vi "SLL DE Group Device Based on Catagory.vi"(8 "error Input":errorcluster, 9 "Module Dev Names":cluster{"Chassis.ModuleDevNames":tag[]}[](array[cluster]), 10 "Chassis Names":tag[](array[tag]), 11 "Device Names":tag[](array[tag])) -> (0 "error out":errorcluster, 2 "Devices Names":string[](array[string]), 3 "All Device Names (Chassis & Module)":cluster{"New element":tag[]}[](array[cluster]))   [LabVIEW 2013]
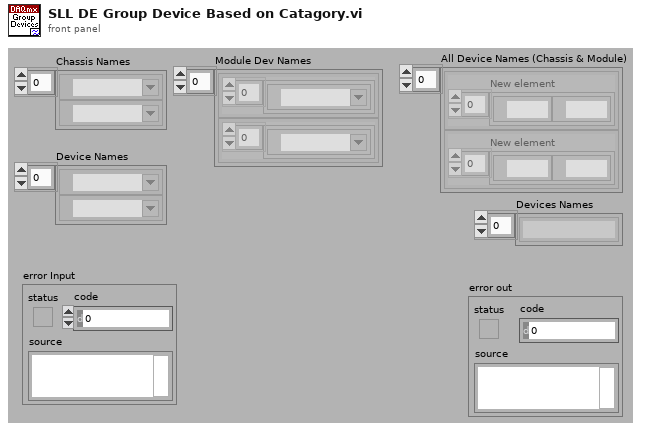
[diagram p1: front panel]
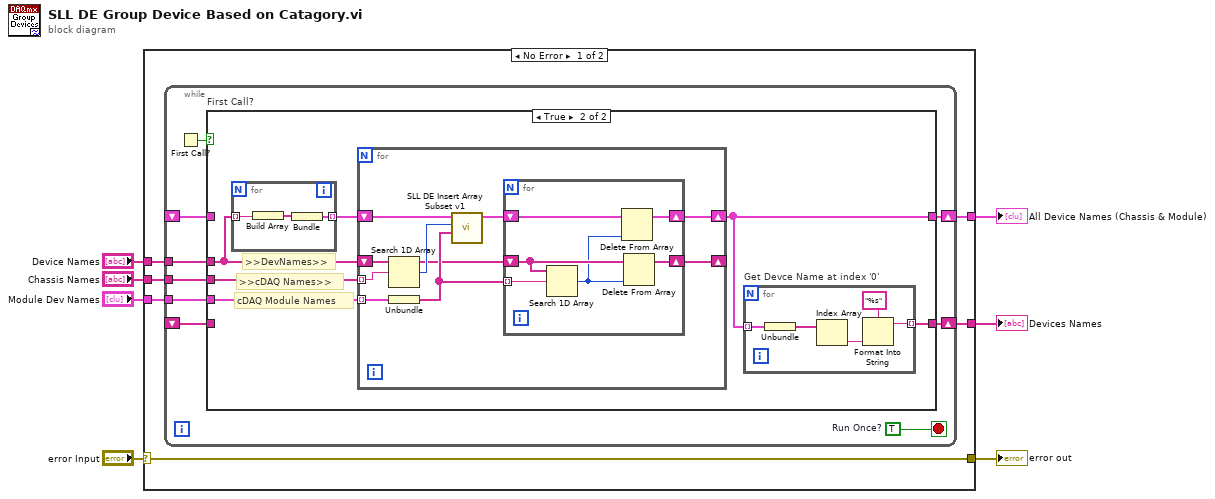
[diagram p0: block diagram]
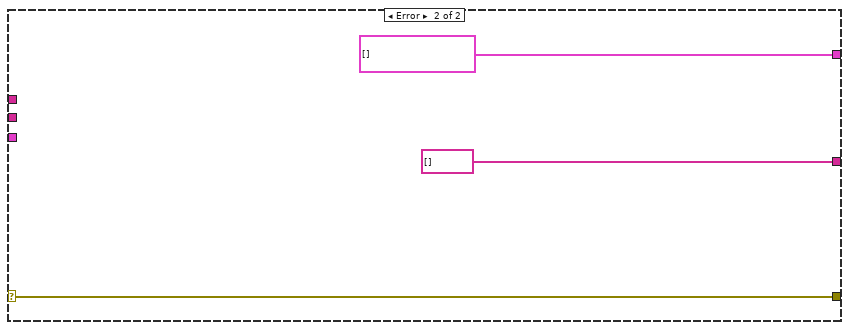
[diagram p3: hidden frame]
diagram:
  n1 = case shown="No Error" "error Input" {
    selector: "error Input" -> [w9 w56]
    tunnel: [w13 cluster{tag[]}[] []] -> w2
    tunnel: "Module Dev Names" -> [w12 _]
    tunnel: "Chassis Names" -> [w11 _]
    tunnel: "Device Names" -> [w10 _]
    tunnel: [w9 w56] -> w3
    tunnel: [w8 string[] []] -> w1
    frame No Error {
      n2 = while {
        tunnel: w12 -> [w21]
        tunnel: w11 -> [w20]
        tunnel: w10 -> [w19]
        shift-right: [w22] -> w13
        shift-left: _ -> [w17]
        shift-right: [w15] -> w8
        shift-left: _ -> [w14]
        stop <- w18 stop-if-true
        w18 = TRUE  # Run Once?
        n3 = First Call?() -> (First Call?: T/F=w16:bool)
        n4 = case "First Call?" shown="True" w16 {
          tunnel: [w24 w26] -> w22
          tunnel: w21 -> [_ w30]
          tunnel: w20 -> [_ w29]
          tunnel: w19 -> [_ w28]
          tunnel: w17 -> [w24 _]
          tunnel: [w23 w25] -> w15
          tunnel: w14 -> [w23 _]
          frame False {
          }
          frame True {
            # "cDAQ Module Names"
            # ">>cDAQ Names>>"
            # ">>DevNames>>"
            n5 = for {
              tunnel: w28 -> [w38] mode=indexing
              tunnel: [w36] -> w27 mode=indexing
              n6 = Build Array(w38) -> (w37:tag[])
              n7 = Bundle(w37) -> (w36:cluster{tag[]})  [unwired: 1 in]
            }
            n8 = for {
              tunnel: w29 -> [w47] mode=indexing
              tunnel: w30 -> [w44] mode=indexing
              shift-right: [w39] -> w26
              shift-left: w27 -> [w46]
              shift-right: [w41] -> _
              shift-left: w28 -> [w42]
              n9 = Search 1D Array(1D array=w42, element=w47) -> (index of element=w45:i32)  [unwired: 1 in]
              n10 = Unbundle(w44) -> ("Chassis.ModuleDevNames"=w43:tag[])
              n11 = call "SLL DE Insert Array Subset v1.vi"("New element"=w43, "Channel index"=w45, "Channel Name"=w46) -> ("Channel Name"=w40:cluster{"New element":tag[]}[])  [unwired: 7 in, 1 out]
              n12 = for {
                tunnel: w43 -> [w53] mode=indexing
                shift-right: [w48] -> w39
                shift-left: w40 -> [w49]
                shift-right: [w51] -> w41
                shift-left: w42 -> [w52]
                n13 = Search 1D Array(1D array=w52, element=w53) -> (index of element=w50:i32)  [unwired: 1 in]
                n14 = Delete From Array(array=w49, index=w50) -> (array with subset deleted=w48:cluster{"New element":tag[]}[])  [unwired: 1 in, 1 out]
                n15 = Delete From Array(array=w52, index=w50) -> (array with subset deleted=w51:tag[])  [unwired: 1 in, 1 out]
              }
            }
            n16 = for "Get Devce Name at index '0'" {
              tunnel: w26 -> [w35] mode=indexing
              tunnel: [w31] -> w25 mode=indexing
              n17 = Unbundle(w35) -> (w34:tag[])
              n18 = Index Array(array=w34) -> (element=w33:tag)  [unwired: 1 in]
              n19 = Format Into String(format string="%s", w33) -> (resulting string=w31:string)  [unwired: 2 in, 1 out]
            }
          }
        }
      }
    }
    frame Error {
    }
  }
  "All Device Names (Chassis & Module)" <- w2
  "error out" <- w3
  "Devices Names" <- w1
